vi "Configure Acquisition Record Core.vi"(0 "IVI_Scope in":refnum<class "IVI_Scope.lvclass">, 5 "time per record (1.0E-3 s)":dbl[unit]=0.001 format="%^.2e", 7 "min record length (100 samples)":i32=100, 9 "acquisition start time (0.0 s)":dbl[unit] format="%.3f", 11 "error in (no error)":errorcluster) -> (4 "IVI_Scope out":refnum<class "IVI_Scope.lvclass">, 15 "error out":errorcluster)   [LabVIEW 2015, in "IVI_Scope.lvlib" / "IVI_Scope.lvclass"]
doc: "This VI configures the most commonly configured properties of the oscilloscope acquisition subsystem. These properties are the time per record, minimum record length, and the acquisition start time."
uses:
  IVI_Scope.lvclass
  IVI_Scope.lvclass/IVI_Scope.ctl
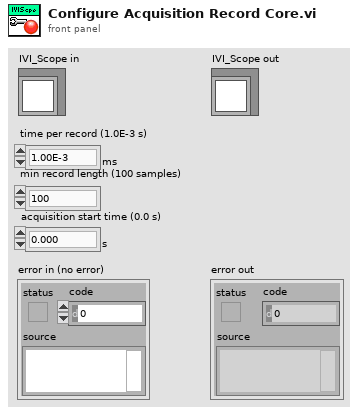
[diagram p1: front panel]
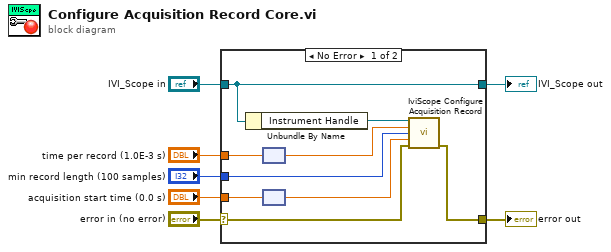
[diagram p0: block diagram]
diagram:
  n1 = case shown="No Error" "error in (no error)" {
    selector: "error in (no error)" -> [w14 w18]
    tunnel: [w13 w18] -> w6
    tunnel: [w16 w17] -> w4
    tunnel: "IVI_Scope in" -> [w16 w17]
    tunnel: "time per record (1.0E-3 s)" -> [w8 _]
    tunnel: "min record length (100 samples)" -> [w12 _]
    tunnel: "acquisition start time (0.0 s)" -> [w11 _]
    frame No Error {
      n2 = Unbundle By Name(w16) -> ("Instrument Handle"=w15:refnum<k15>)
      n3 = node(w8) -> (w10:dbl)
      n4 = node(w11) -> (w9:dbl)
      n5 = call <vilib>:"IviScope Configure Acquisition Record.vi"("instrument handle"=w15, "time per record (1.0E-3 s)"=w10, "min record length (100 samples)"=w12, "acquisition start time (0.0 s)"=w9, "error in (no error)"=w14) -> ("error out"=w13:errorcluster)  [unwired: 9 in, 1 out]
    }
    frame Error {
    }
  }
  "error out" <- w6
  "IVI_Scope out" <- w4
